vi "Configure Analog Still Output.vi"(0 "VISA resource name":refnum<visa-resource-name>, 1 "Analog Out Mode (0: Off)":u16(ring) items=["Off"=0, "Monitor Out"=1, "Open Loop (Manual)"=2, "Still"=4], 2 "Source (1: Kelvin)":u16(ring)=1 items=["Kelvin"=1, "Ohms"=2], 3 "Enable Bipolar Mode (F: Disable)":bool, 5 "Channel (1:1)":u16(ring)=1 items=["none", "1", "2", "3", "4", "5", "6", "7", "8", "9", "10", "11", "12", "13", "14", "15", "16", "A (Control Input)"], 7 "High Value (0.00000E+0)":dbl min=0.0 max=100.0 step=1e-06 format="%^.5e", 9 "Low Value (0.00000E+0)":dbl min=-100.0 max=100.0 step=1e-06 format="%^.5e", 11 "error in (no error)":errorcluster, 12 "Manual Value (0.000%)":dbl min=-100.0 max=100.0 step=0.001 format="%.3f", 13 "Still Value (0.000%)":dbl min=-100.0 max=100.0 step=0.001 format="%.3f") -> (4 "VISA resource name out":refnum<visa-resource-name>, 15 "error out":errorcluster)   [LabVIEW 2018, in "Lake Shore 372.lvlib"]
doc: "Configures the 372 analog(still) output. The Model 372 has one analog voltage output that is designated as ANALOG OUT 2 (STILL). It is a variable DC voltage source that can vary from +10V to -10V\n\nNotes:\nWhen possible, it is recommended to use the <B>OUTMODE</B> command to configure both the warm-up heater and the analog/still output."
uses:
  Lake Shore 372.lvlib
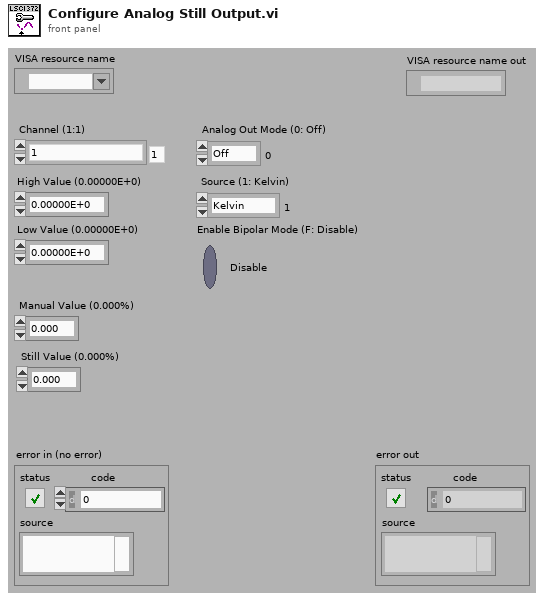
[diagram p1: front panel]
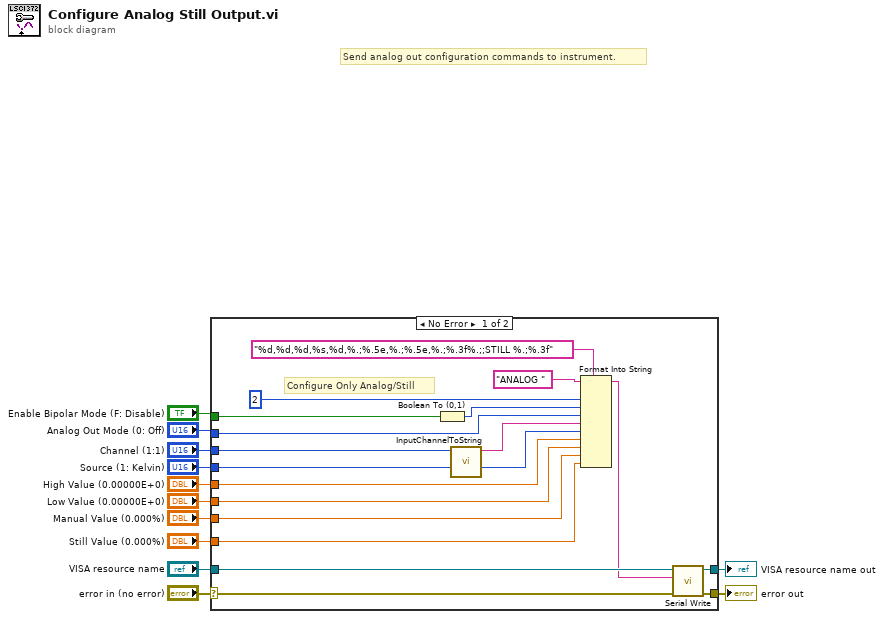
[diagram p0: block diagram]
diagram:
  # "Send analog out configuration commands to instrument."
  n1 = case shown="No Error" "error in (no error)" {
    selector: "error in (no error)" -> [w22 w31]
    tunnel: "VISA resource name" -> [w30 w32]
    tunnel: [w29 w31] -> w11
    tunnel: [w28 w32] -> w10
    tunnel: "Still Value (0.000%)" -> [w25 _]
    tunnel: "Enable Bipolar Mode (F: Disable)" -> [w20 _]
    tunnel: "Analog Out Mode (0: Off)" -> [w19 _]
    tunnel: "Channel (1:1)" -> [w18 _]
    tunnel: "Source (1: Kelvin)" -> [w17 _]
    tunnel: "High Value (0.00000E+0)" -> [w16 _]
    tunnel: "Low Value (0.00000E+0)" -> [w15 _]
    tunnel: "Manual Value (0.000%)" -> [w14 _]
    frame No Error {
      # "Configure Only Analog/Still"
      n2 = Boolean To (0,1)(Boolean=w20) -> (0, 1=w26:i16)
      n3 = call "InputChannelToString.vi"("Channel (1)"=w18) -> ("Channel Str"=w23:string)  [unwired: 10 in]
      n4 = Format Into String(format string="%d,%d,%d,%s,%d,%.;%.5e,%.;%.5e,%.;%.3f%.;;STILL %.;%.3f", initial string="ANALOG ", u16 2 ("input 1"), w26, w19, w23, w17, w16, w15, w14, w25) -> (resulting string=w24:string)  [unwired: 1 in, 1 out]
      n5 = call "Serial Write.vi"("error in (no error)"=w22, "Write Buffer (\"\")"=w24, "VISA resource name"=w30) -> ("error out"=w29:errorcluster, "VISA resource name out"=w28:refnum<visa-resource-name>)  [unwired: 6 in, 1 out]
    }
    frame Error {
    }
  }
  "error out" <- w11
  "VISA resource name out" <- w10
